vi "Data_send.vi"(6 "Full Scale":sgl, 7 "Start_communication":bool, 8 "error in (no error)":errorcluster, 9 "Relative Motor position PLC":dbl, 10 "Direction":bool, 11 "VISA resource name":refnum<visa-resource-name>) -> (0 "Retransmission count":i32, 1 "Motor ready":bool, 2 "PLC error out":errorcluster, 3 "Arduino error out":errorcluster, 4 "VISA resource name out":refnum<visa-resource-name>, 5 "Communication Acnowledge":bool)   [LabVIEW 2018]
uses:
  <vilib>/OPCUA/controls/NodeId.ctl
  Main_SubVI/Progress.vi
  <vilib>/OPCUA/NI OPC UA Client.lvlib
panel:
  out "read buffer 2":string
  out "Relative Motor position Arduino 2":dbl
  out "Data Info":string
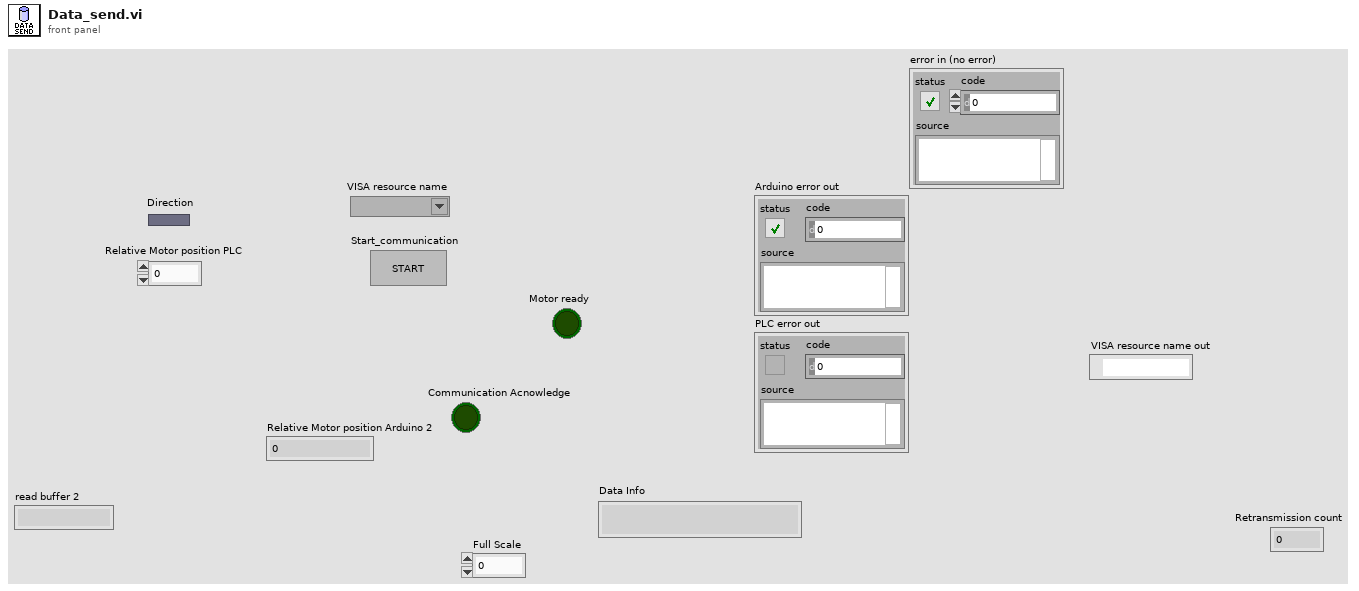
[diagram p1: front panel]
types:
  T1 = cluster{"message mode":enum16{"None", "Sign", "Sign and Encrypt"}, "security":enum16{"Basic256", "Basic128Rsa15"}}
  T2 = typedef "OPC UA Client Refnum.ctl" = refnum<k21>
  T3 = typedef "NodeId.ctl" = string
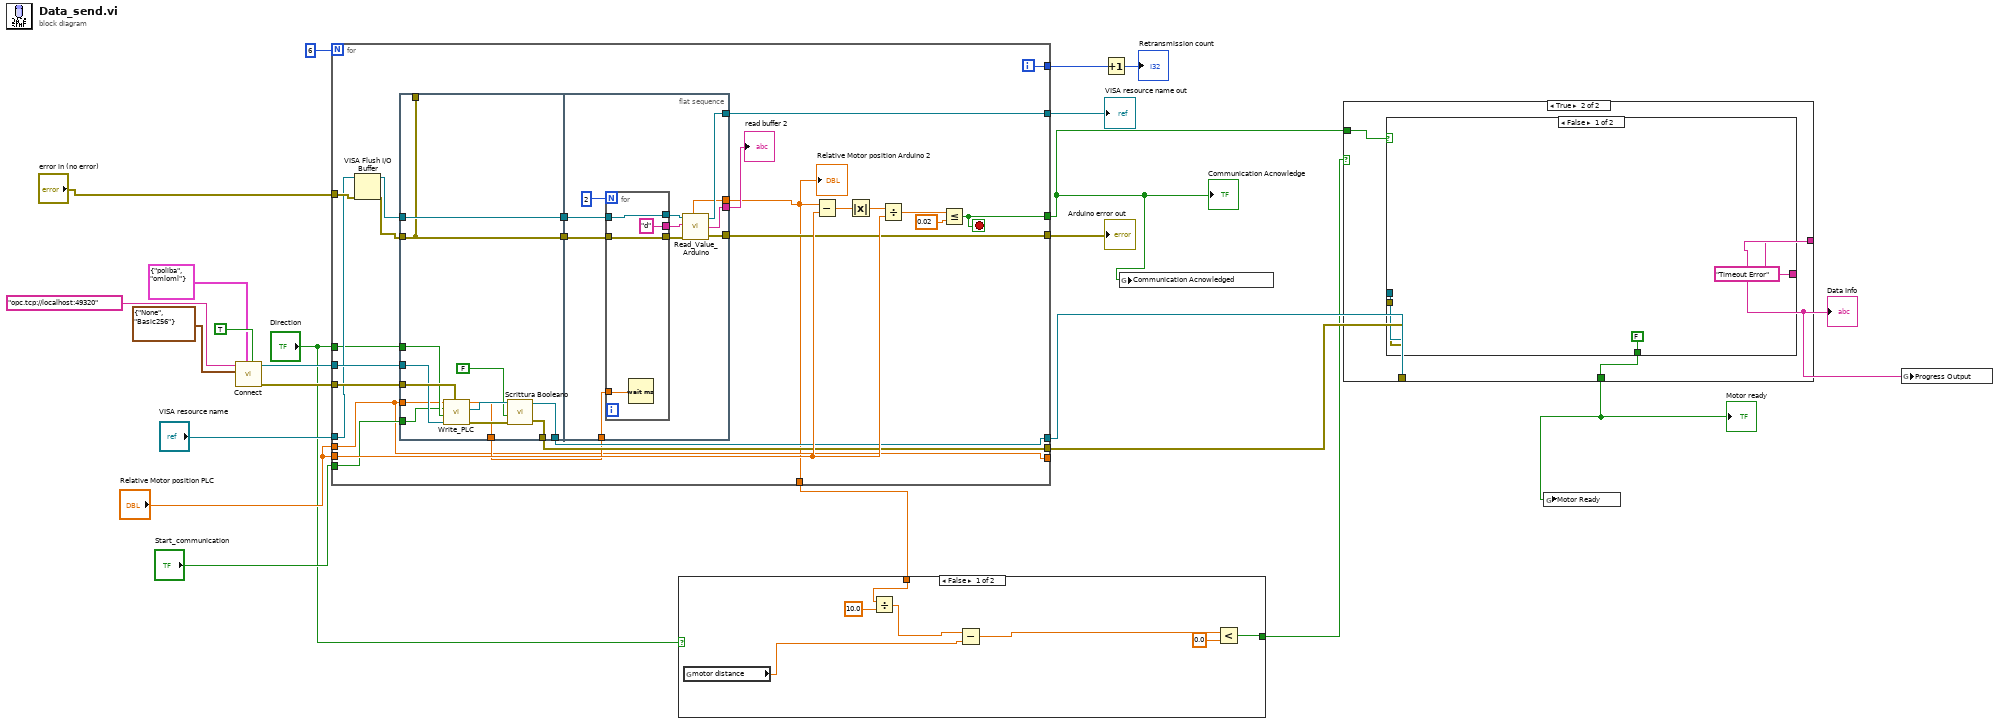
[diagram p0: block diagram]
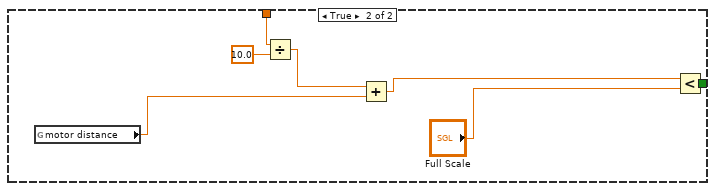
[diagram p2: hidden frame]
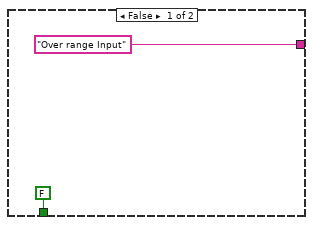
[diagram p3: hidden frame]
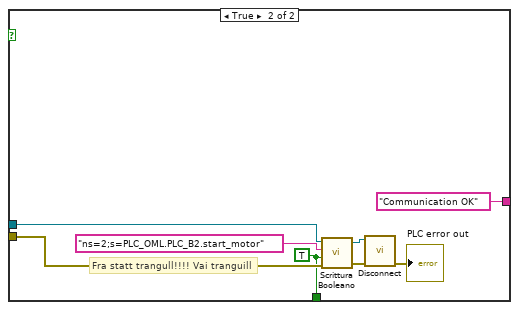
[diagram p4: hidden frame]
diagram:
  n1 = call <vilib>:"Connect.vi"("trust any server (F)"=TRUE, "username/password"=cluster{"username":string, "password":string} {"username"="poliba", "password"="omloml"}, "security policy"=T1 {"message mode"=enum."None", "security"=enum."Basic256"}, "server endpoint URL"="opc.tcp://localhost:49320") -> ("error out"=w16:errorcluster, "OPC UA client refnum out"=w17:T2)  [unwired: 5 in, 1 out]
  n2 = for {
    N: 6 -> [_]
    tunnel: [w48] -> w18
    tunnel: w17 -> [w38]
    tunnel: "Direction" -> [w24]
    tunnel: "Relative Motor position PLC" -> [w30]
    tunnel: "Start_communication" -> [w37]
    tunnel: w16 -> [w39]
    tunnel: [w34] -> w11
    tunnel: "Relative Motor position PLC" -> [w43]
    tunnel: [w41] -> w9
    tunnel: [w40] -> w8
    tunnel: [w45] -> w6
    tunnel: [w32] -> w12
    tunnel: "VISA resource name" -> [w25]
    tunnel: [w30] -> _
    tunnel: [w29] -> w2
    tunnel: "error in (no error)" -> [w28]
    i -> [w48]
    stop <- w45 stop-if-true
    n3 = VISA Flush I/O Buffer(VISA resource name=w25, error in (no error)=w28) -> (VISA resource name out=w26:refnum<visa-resource-name>, error out=w27:errorcluster)  [unwired: 1 in]
    n4 = flat-sequence {
      tunnel: [w61] -> w41
      tunnel: [w60] -> w40
      tunnel: w39 -> [w59]
      tunnel: w38 -> [w58]
      tunnel: w24 -> [w57]
      tunnel: w37 -> [w56]
      tunnel: w30 -> [w55]
      tunnel: [w52] -> w31
      tunnel: w26 -> [w50]
      tunnel: [w49] -> _
      tunnel: [w50] -> w36
      tunnel: [w49] -> w35
      tunnel: w27 -> [w49]
      tunnel: w31 -> [w72]
      tunnel: w36 -> [w70]
      tunnel: w35 -> [w71]
      tunnel: [w68] -> w34
      tunnel: [w67] -> w33
      tunnel: [w66] -> w32
      tunnel: [w62] -> w29
      frame #0 {
        n5 = call "Write_PLC.vi"("error in"=w59, "OPC UA client refnum out"=w58, "Direction"=w57, "Start_communication"=w56, "Relative_Motor_position"=w55) -> ("error out"=w54:errorcluster, "OPC UA client refnum out 2"=w53:T2, "recommended delay"=w52:dbl)  [unwired: 1 out]
        n6 = call "Scrittura Booleano.vi"("OPC UA client refnum in"=w53, "Value"=FALSE, "error in (no error)"=w54) -> ("OPC UA client refnum out"=w61:T2, "error out"=w60:errorcluster)  [unwired: 2 in, 1 out]
      }
      frame #1 {
        n7 = for {
          N: 2 -> [_]
          tunnel: w72 -> [w76]
          tunnel: ["d" ("write buffer")] -> w69
          tunnel: w71 -> [w73]
          tunnel: w70 -> [w74]
          tunnel: [w74] -> w65
          tunnel: [w73] -> w64
          n8 = Wait (ms)(milliseconds to wait=w76) -> ()  [unwired: 1 out]
        }
        n9 = call "Read_Value_Arduino.vi"("VISA resource name"=w65, "write buffer"=w69, "error in (no error)"=w64) -> ("output"=w62:dbl, "VISA resource name out"=w66:refnum<visa-resource-name>, "concatenated string"=w67:string, "error out"=w68:errorcluster)  [unwired: 1 in]
      }
    }
    n10 = Subtract(x=w29, y=w43) -> (x-y=w46:dbl)
    n11 = Absolute Value(x=w46) -> (abs(x)=w44:dbl)
    n12 = Divide(x=w44, y=w43) -> (x/y=w42:dbl)
    n13 = Less Or Equal?(x=w42, y=0.02) -> (x <= y?=w45:bool)
    "read buffer 2" <- w33
    "Relative Motor position Arduino 2" <- w29
  }
  "Arduino error out" <- w11
  "VISA resource name out" <- w12
  "Communication Acnowledge" <- w6
  n14 = case shown="False" "Direction" {
    tunnel: w2 -> [w82 w85]
    tunnel: [w79 w84] -> w1
    frame False {
      n15 = global read "Progress.vi" "motor distance"() -> (w80:dbl)
      n16 = Divide(x=w82, y=10.0) -> (x/y=w81:dbl)
      n17 = Subtract(x=w81, y=w80) -> (x-y=w78:dbl)
      n18 = Less?(x=w78, y=0.0) -> (x < y?=w79:bool)
    }
    frame True {
      n19 = global read "Progress.vi" "motor distance"() -> (w88:dbl)
      n20 = Divide(x=w85, y=10.0) -> (x/y=w89:dbl)
      n21 = Add(x=w89, y=w88) -> (x+y=w90:dbl)
      n22 = Less?(x=w90, y="Full Scale") -> (x < y?=w84:bool)
    }
  }
  n23 = Increment(x=w18) -> (x+1=→"Retransmission count":i32)
  n24 = global write "Progress.vi" "Communication Acnowledged"(w6) -> ()
  n25 = case shown="True" w1 {
    tunnel: w6 -> [_ w97]
    tunnel: w9 -> [_ w96]
    tunnel: w8 -> [_ w95]
    tunnel: ["Over range Input" ("Data Info") w94] -> w4
    tunnel: [FALSE ("Value") w93] -> w7
    frame False {
    }
    frame True {
      n26 = case shown="False" w97 {
        tunnel: w96 -> [_ w106]
        tunnel: w95 -> [_ w104]
        tunnel: ["Timeout Error" ("Data Info") "Communication OK" ("Data Info 2")] -> w94
        tunnel: [FALSE ("Value") w100] -> w93
        frame False {
        }
        frame True {
          w100 = TRUE ("Value")
          # "Fra statt trangull!!!! Vai tranguill"
          n27 = call "Scrittura Booleano.vi"("OPC UA client refnum in"=w106, "node ID"=T3 "ns=2;s=PLC_OML.PLC_B2.start_motor", "Value"=w100, "error in (no error)"=w104) -> ("OPC UA client refnum out"=w103:T2, "error out"=w102:errorcluster)  [unwired: 1 in, 1 out]
          n28 = call <vilib>:"Disconnect.vi"("error in (no error)"=w102, "OPC UA client refnum in"=w103) -> ("error out"=→"PLC error out":errorcluster)  [unwired: 9 in]
        }
      }
    }
  }
  "Data Info" <- w4
  "Motor ready" <- w7
  n29 = global write "Progress.vi" "Motor Ready"(w7) -> ()
  n30 = global write "Progress.vi" "Progress Output"(w4) -> ()
